vi "InsertMenubarItem.vi"(6 "Insert After (last)":i32, 8 "error in (no error)":errorcluster, 9 "Sub Items":T1(array[cluster]), 10 "Menu Name":string, 11 "menu ref":refnum<k9>) -> (0 "error out":errorcluster, 1 "Sub Item Tags":string[](array[string]), 2 "Menu Tag":string, 3 "menu ref out":refnum<k9>, 4 "Sub Item Names":string[](array[string]))   [LabVIEW 2019]
uses:
  <vilib>/Utility/miscctls.llb/LVMenuShortCut.ctl
panel:
  # "アクセスキーの指定は直前に _ を置く"
  # "セパレータは APP_SEPARATOR"
  # "先頭に置くには -1\n2番目に入れるなら 0\n大きすぎれば末尾"
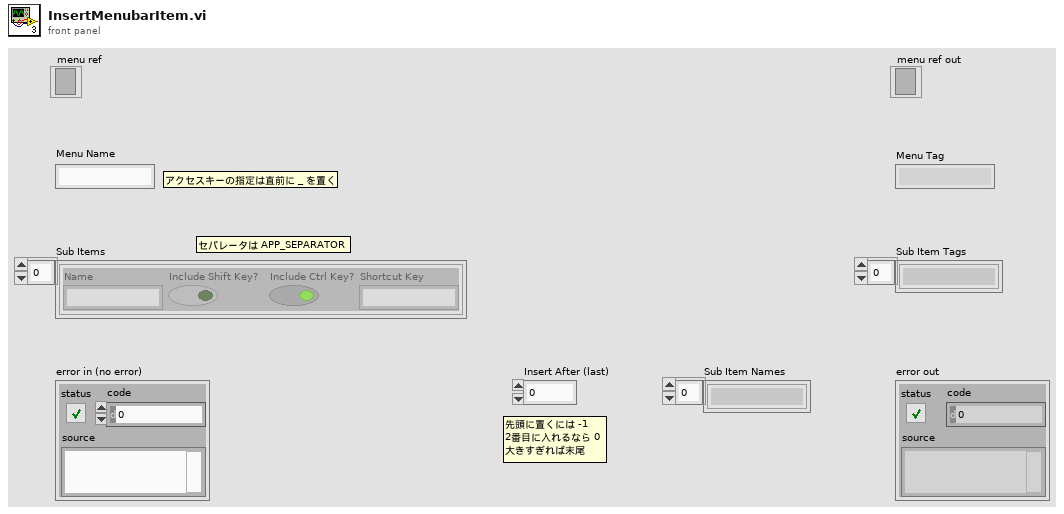
[diagram p1: front panel]
types:
  T1 = cluster{"Name":string, "Include Shift Key?":bool, "Include Ctrl Key?":bool, "Shortcut Key":string}[]
  T2 = typedef "LVMenuShortCut.ctl" = cluster{"Include Shift Key?":bool, "Include Ctrl Key?":bool, "Shortcut Key":string}
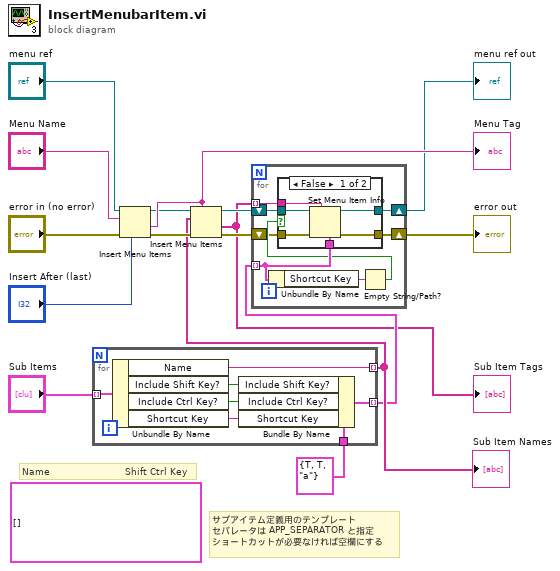
[diagram p0: block diagram]
diagram:
  (unwired) T1 [] ("Menu Short Cut")
  # "Name                         Shift Ctrl Key"
  # "サブアイテム定義用のテンプレート\nセパレータは APP_SEPARATOR と指定\nショートカットが必要なければ空欄にする"
  n1 = for {
    tunnel: "Sub Items" -> [w23] mode=indexing
    tunnel: [w22] -> w9 mode=indexing
    tunnel: [w18] -> w7 mode=indexing
    tunnel: T2 {"Include Shift Key?"=TRUE, "Include Ctrl Key?"=TRUE, "Shortcut Key"="a"} ("Menu Short Cut") -> [w17]
    n2 = Unbundle By Name(w23) -> ("Name"=w22:string, "Include Shift Key?"=w21:bool, "Include Ctrl Key?"=w20:bool, "Shortcut Key"=w19:string)
    n3 = Bundle By Name(cluster=w17, "Include Shift Key?"=w21, "Include Ctrl Key?"=w20, "Shortcut Key"=w19) -> (w18:T2)
  }
  "Sub Item Names" <- w9
  n4 = Insert Menu Items(4:"Insert After (last)", 6:"error in (no error)", 8:"Menu Name", 9:"menu ref") -> (0:w10:errorcluster, 1:w12:string, 3:w11:refnum<k9>)  [unwired: 2 in]
  "Menu Tag" <- w12
  n5 = Insert Menu Items(5:w12, 6:w10, 8:w9, 9:w11) -> (0:w6:errorcluster, 1:w3:string[], 3:w8:refnum<k9>)  [unwired: 2 in]
  "Sub Item Tags" <- w3
  n6 = for {
    tunnel: w3 -> [w31] mode=indexing
    tunnel: w7 -> [w30] mode=indexing
    shift-right: [w26] -> w4
    shift-left: w8 -> [w27]
    shift-right: [w24] -> w2
    shift-left: w6 -> [w25]
    n7 = Unbundle By Name(w30) -> ("Shortcut Key"=w29:string)
    n8 = Empty String/Path?(string/path=w29) -> (empty?=w28:bool)
    n9 = case shown="False" w28 {
      tunnel: w31 -> [w37 _]
      tunnel: w30 -> [w36 _]
      tunnel: w27 -> [w35 w39]
      tunnel: [w34 w39] -> w26
      tunnel: w25 -> [w33 w38]
      tunnel: [w32 w38] -> w24
      frame False {
        n10 = Set Menu Item Info(4:w36, 7:w37, 8:w33, 11:w35) -> (0:w32:errorcluster, 3:w34:refnum<k9>)  [unwired: 3 in]
      }
      frame True {
      }
    }
  }
  "menu ref out" <- w4
  "error out" <- w2
